vi "Configure Voltage.vi"(8 "error in (no error)":errorcluster, 10 "Voltage":dbl, 11 "Keithley 24xx in":refnum<class "Keithley 24xx.lvclass">) -> (0 "error out":errorcluster, 3 "Keithley 24xx out":refnum<class "Keithley 24xx.lvclass">)   [LabVIEW 2020, in "Keithley 24xx.lvclass"]
uses:
  Keithley 24xx.lvclass
  C:/Sandbox/Git_Sandbox/WiSpry Test Framework source code (LV20)/WiSpry Test Framework/Instruments/Instrument.lvclass
  C:/Sandbox/Git_Sandbox/WiSpry Test Framework source code (LV20)/WiSpry Test Framework/Instruments/Power Supply/Power Supply.lvclass
  Instrument.lvclass/Instrument.ctl
  Power Supply.lvclass/Power Supply.ctl
  Instrument.lvclass
  <instrlib>/Keithley 24XX/Keithley 24XX.lvlib
  Power Supply.lvclass
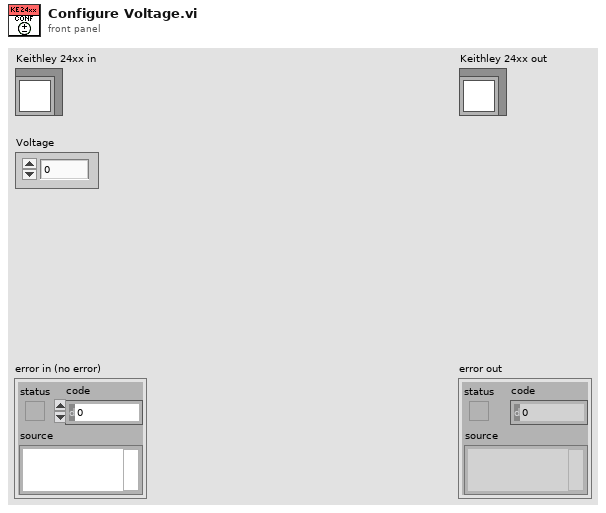
[diagram p1: front panel]
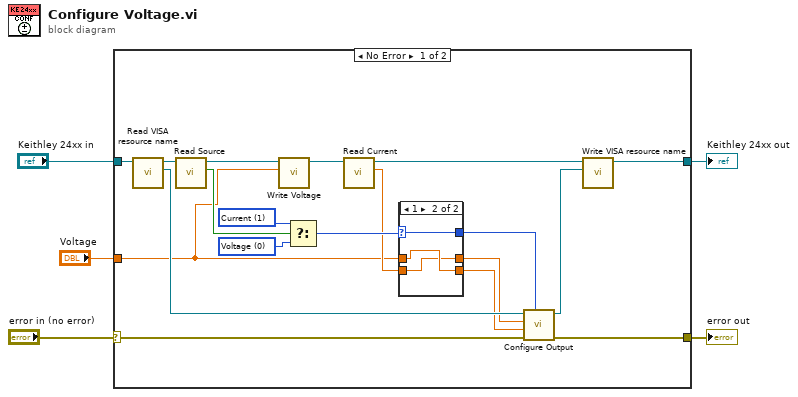
[diagram p0: block diagram]
diagram:
  n1 = case shown="No Error" "error in (no error)" {
    selector: "error in (no error)" -> [w22 w32]
    tunnel: [w21 w32] -> w5
    tunnel: [w23 w31] -> w4
    tunnel: "Keithley 24xx in" -> [w24 w31]
    tunnel: "Voltage" -> [w6 _]
    frame No Error {
      w16 = u16 0 items=["Voltage", "Current"] ("Source Mode  (0: Voltage)")
      w17 = u16 1 items=["Voltage", "Current"] ("Source Mode  (0: Voltage)")
      n2 = call "Read VISA resource name.vi"("Instrument in"=w24) -> ("VISA resource name"=w19:refnum<visa-resource-name>, "Instrument out"=w13:refnum<class "Keithley 24xx.lvclass">)  [unwired: 9 in]
      n3 = call-dynamic "Read Source.vi"("Power Supply in"=w13) -> ("Source"=w18:bool, "Power Supply out"=w8:refnum<class "Keithley 24xx.lvclass">)  [unwired: 9 in]
      n4 = call "Write Voltage.vi"("Voltage"=w6, "Power Supply in"=w8) -> ("Power Supply out"=w7:refnum<class "Keithley 24xx.lvclass">)  [unwired: 9 in]
      n5 = Select(t=w17, s=w18, f=w16) -> (s? t:f=w15:u16)
      n6 = call "Read Current.vi"("Power Supply in"=w7) -> ("Current"=w11:dbl, "Power Supply out"=w12:refnum<class "Keithley 24xx.lvclass">)  [unwired: 9 in]
      n7 = case shown="1" w15 {
        selector: w15 -> [w26 w29]
        tunnel: [w27 w28] -> w14
        tunnel: w6 -> [w27 w30]
        tunnel: w11 -> [w25 w28]
        tunnel: [w25 w30] -> w10
        tunnel: [w26 w29] -> w9
        frame 0, Default {
        }
        frame 1 {
        }
      }
      n8 = call <instrlib>:"Configure Output.vi"("Source Mode  (0: Voltage)"=w9, "error in (no error)"=w22, "Compliance  Level (0.1)"=w10, "Output Level (0)"=w14, "VISA resource name"=w19) -> ("error out"=w21:errorcluster, "VISA resource name out"=w20:refnum<visa-resource-name>)  [unwired: 5 in]
      n9 = call "Write VISA resource name.vi"("VISA resource name"=w20, "Instrument in"=w12) -> ("Instrument out"=w23:refnum<class "Keithley 24xx.lvclass">)  [unwired: 9 in]
    }
    frame Error {
    }
  }
  "error out" <- w5
  "Keithley 24xx out" <- w4
